vi "PXI_MultiTrig.vi"() -> ()   [LabVIEW 2018, in "Visualization.lvlib" / "VisualizeSync.lvclass"]
doc: "This VI listens for any measurement data associated with the provided PluginName and displays it to the user for analysis. The display is only suitable for data coming from the RoomAlert Plugin."
uses:
  VisualizeSync.lvclass
  VisualizeBase/VisualizeBase_class/SubVIs/VisualizationOptions.ctl
  <vilib>/Utility/miscctls.llb/LVRectTypeDef.ctl
  <vilib>/event_ctls.llb/usereventprio.ctl
  VisualizeBase/VisualizeBase_class/Requests/VisUserEventType.ctl
  <extravilib>/ChannelInstances/Tag-bool/Write With Abort.vi
  <extravilib>/ChannelInstances/Tag-bool/Read With Abort.vi
  <extravilib>/ChannelInstances/Tag-bool/Instantiate.vi
  <extravilib>/ChannelInstances/Tag-bool/EndpointRead.vi
  <vilib>/Utility/error.llb/Error Cluster From Error Code.vi
  <extravilib>/ChannelInstances/Tag-bool/Endpoint.vi
  <vilib>/ErrorRing/Error Ring.xnode
  <userlib>/NIST/NISTErrorLib/NISTErrorLib.lvlib
  VisualizeBase/VisualizeBase_class/VisualizeBase.lvclass
  <extravilib>/ChannelInstances/Tag-bool.lvlib
  TestClass/Test.lvclass
  Sync/SyncModule/SyncModule.lvlib
  StatusAndLog/VisualizeStatus.lvclass
panel:
  in  "btnPause":bool=TRUE
  in  "INIFilePath":path
  out "VisualizationProperties":T1={"PauseAtStartup"=TRUE, "LogData"=FALSE, "LaunchInSubPanel"=TRUE, "FPMonitor"=0, "FPWindowBounds"={"Left"=0, "Top"=0, "Right"=0, "Bottom"=0}, "MonitorBounds"={"Left"=0, "Top"=0, "Right"=0, "Bottom"=0}}
  in  "ModuleID":i32
  in  "Log Data":bool=TRUE
  in  "btnStop":bool
  in  "btnReset":bool
  in  "btnClearTest":bool
  out "LockStatus":bool
  out "Time Ref Offset (ns)":waveform(dbl)(graph)
  out "ErrorArray":errorcluster[](array[cluster])
  in  "PluginName":string="Sensor.RoomAlert1"
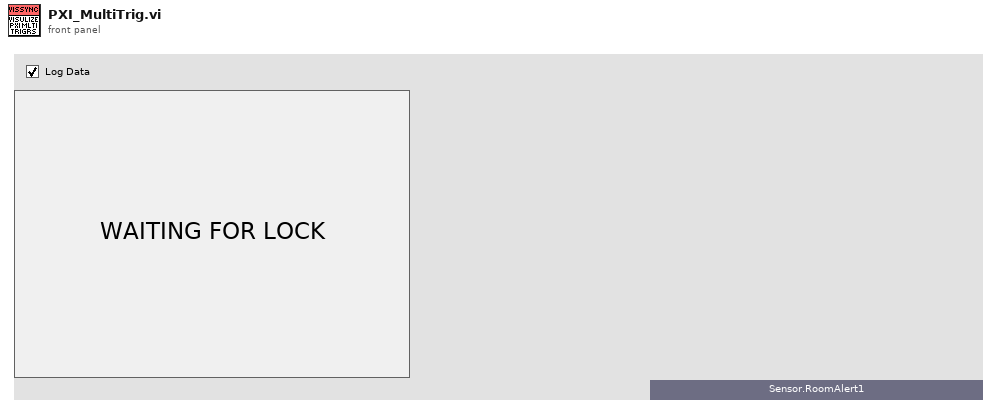
[diagram p1: front panel]
types:
  T1 = typedef "Visualization.lvlib/VisualizeBase.lvclass/VisualizationOptions.ctl" = cluster{"PauseAtStartup":bool, "LogData":bool, "LaunchInSubPanel":bool, "FPMonitor":u16, "FPWindowBounds":T2, "MonitorBounds":cluster{"Left":i16, "Top":i16, "Right":i16, "Bottom":i16}}
  T2 = typedef "LVRectTypeDef.ctl" = cluster{"Left":i16, "Top":i16, "Right":i16, "Bottom":i16}
  T3 = enum16{"open", "open or create", "create or replace", "create", "open (read-only)"}
  T4 = typedef "Visualization.lvlib/VisualizeBase.lvclass/VisRequestEvents.ctl" = cluster{"StopRequest":refnum<user-event>, "ResetRequest":refnum<user-event>, "FP Pop In or Out":refnum<user-event>}
  T5 = typedef "SyncModule.lvlib/SyncBroadcastEvents.ctl" = cluster{"DidInit":refnum<user-event>, "StatusUpdate":refnum<user-event>, "ErrorReport":refnum<user-event>, "DidStop":refnum<user-event>, "PathToINI":refnum<user-event>, "TriggerTime":refnum<user-event>, "LockStatus":refnum<user-event>, "Info":refnum<user-event>, "ClockProperties":refnum<user-event>, "SyncData":refnum<user-event>}
  T6 = cluster{"seconds since 1Jan1904":timestamp, "Time Ref Offset (ns)":dbl, "Lock":bool}
  T7 = typedef "Visualization.lvlib/VisualizeBase.lvclass/VisUserEventType.ctl" = cluster{"BusIndex":i8, "Data":variant}
  T8 = typedef "usereventprio.ctl" = enum32{"high priority", "normal priority"}
  T9 = typedef "Tag-bool.lvlib/))Channel.ctl" = refnum<queue>
  T10 = typedef "sizeaction.ctl" = enum32{"Minimized", "Maximized", "Resized"}
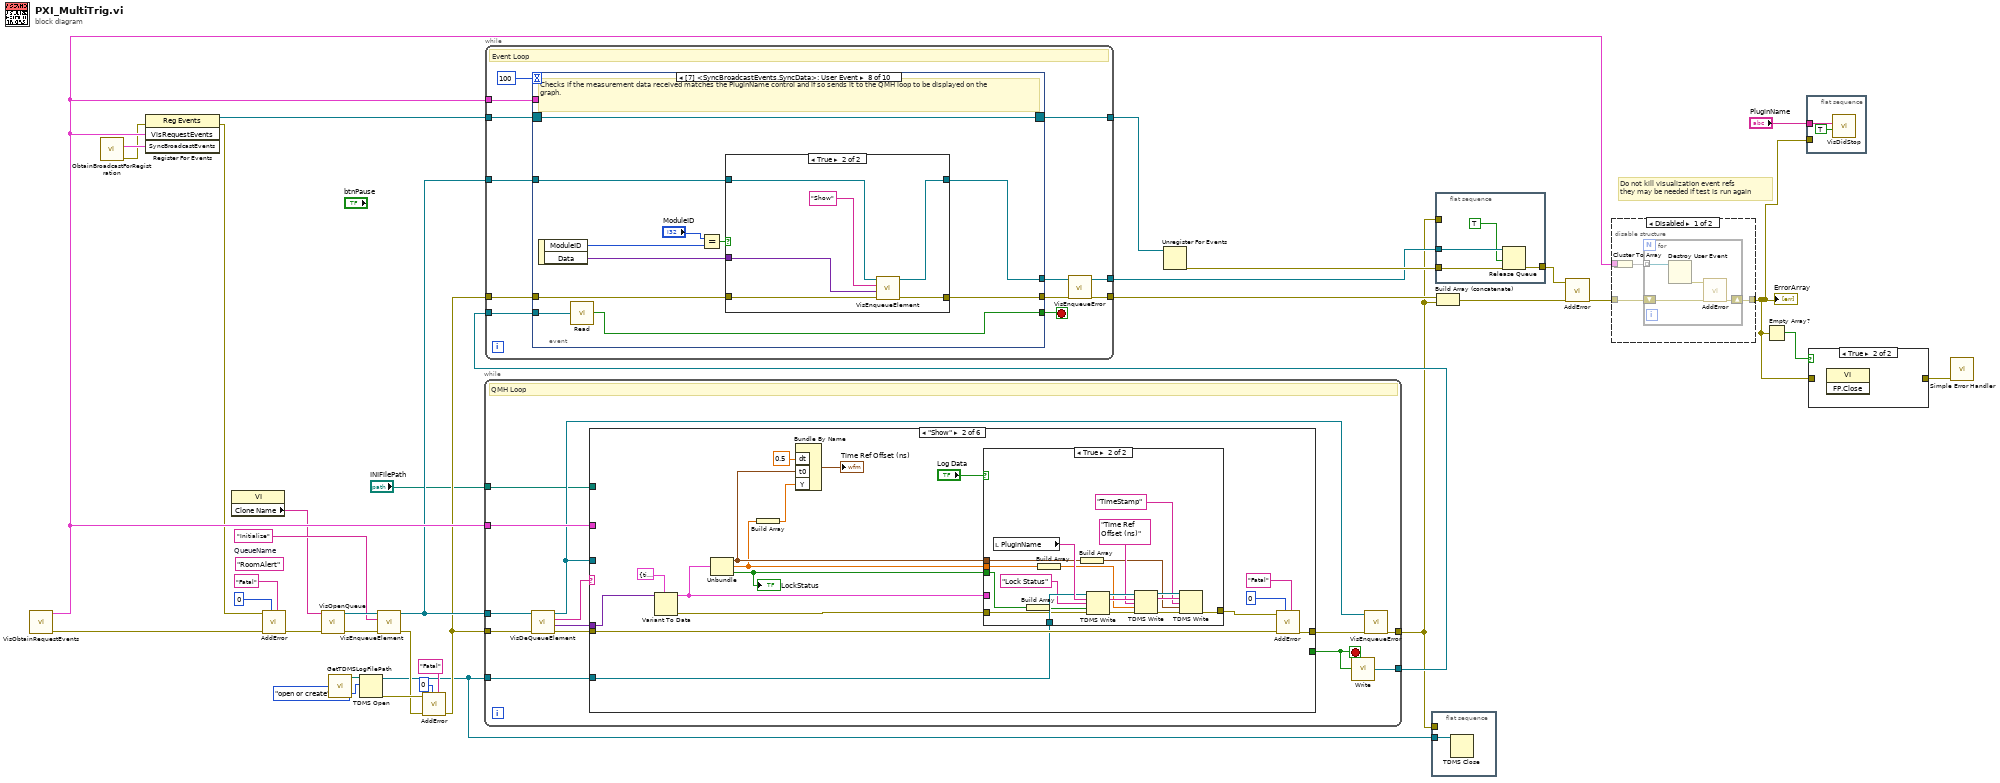
[diagram p0: block diagram]
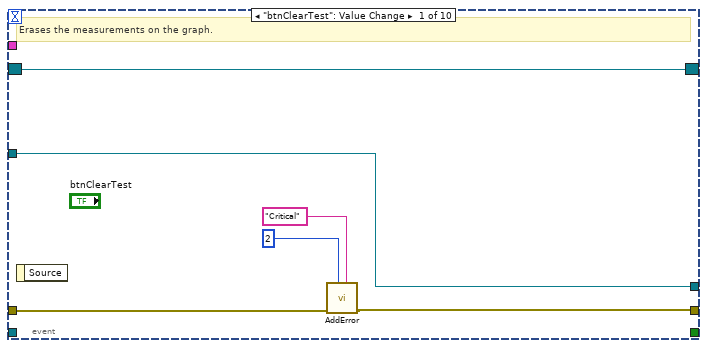
[diagram p3: hidden frame]
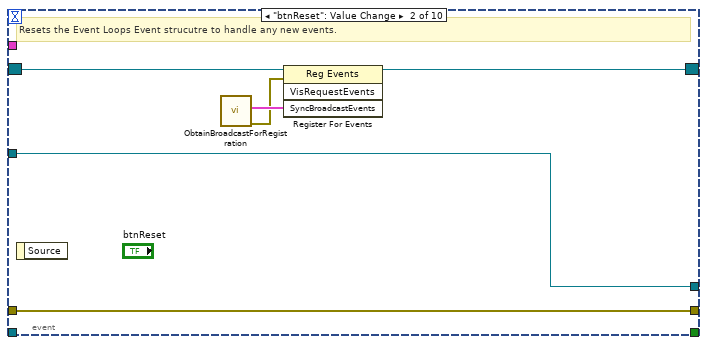
[diagram p4: hidden frame]
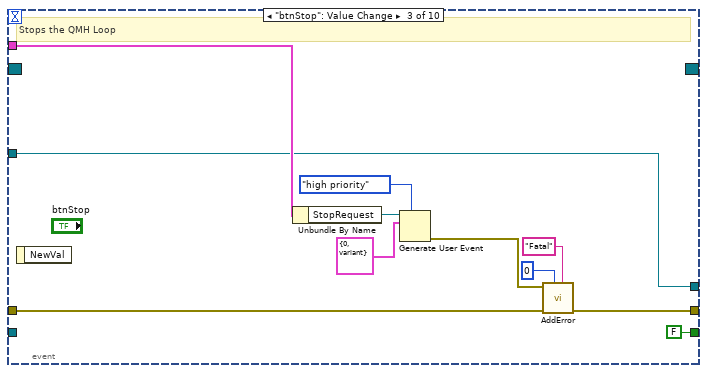
[diagram p5: hidden frame]
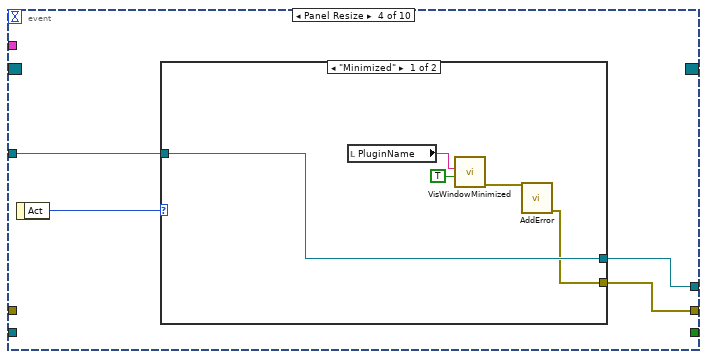
[diagram p6: hidden frame]
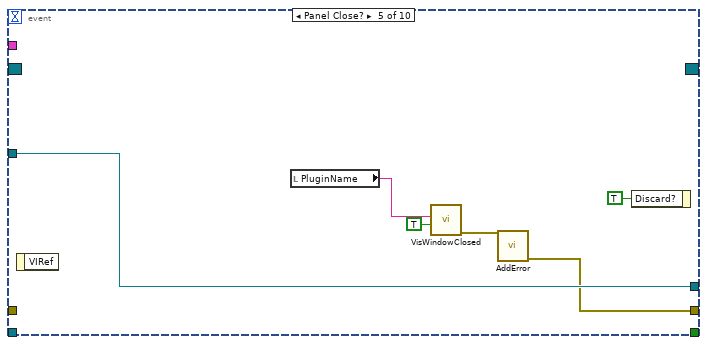
[diagram p8: hidden frame]
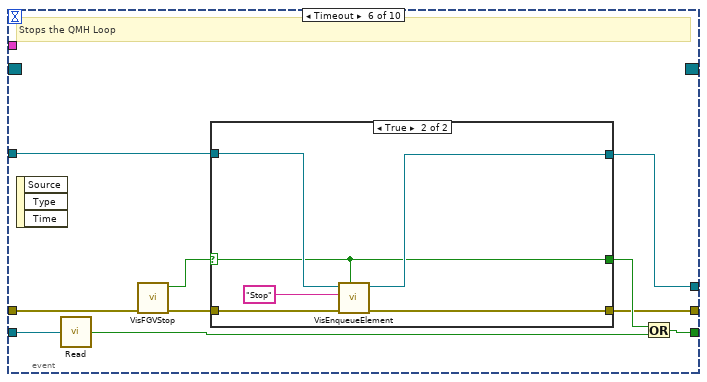
[diagram p9: hidden frame]
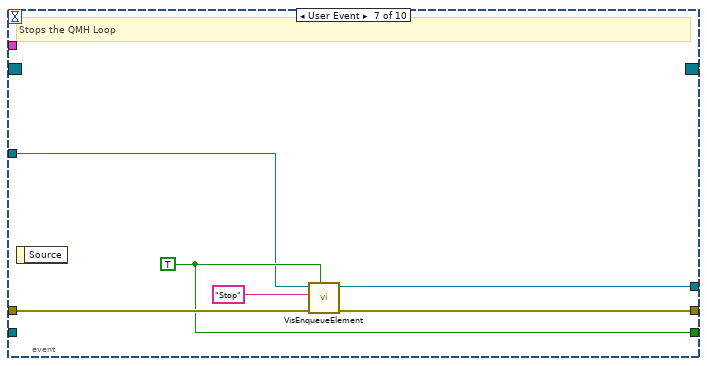
[diagram p11: hidden frame]
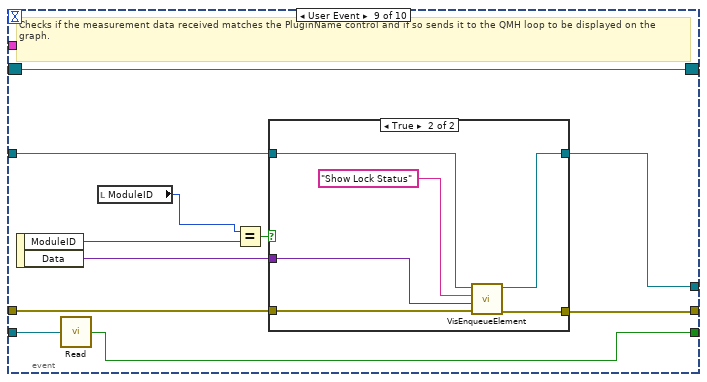
[diagram p13: hidden frame]
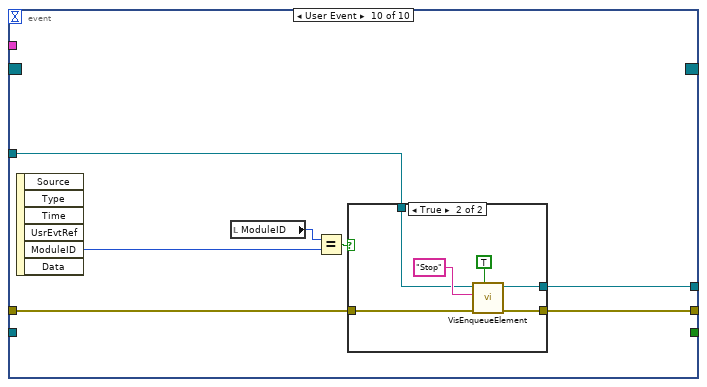
[diagram p15: hidden frame]
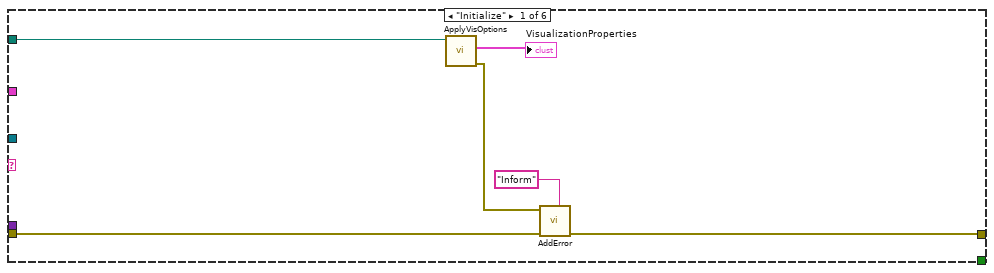
[diagram p17: hidden frame]
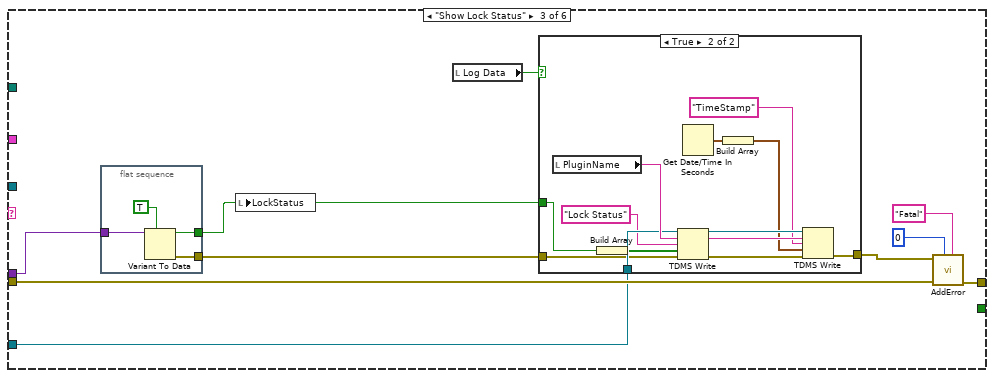
[diagram p19: hidden frame]
diagram:
  (unwired) "RoomAlert"  # QueueName
  # "Do not kill visualization event refs\nthey may be needed if test is run again"
  n1 = call "VisObtainRequestEvents.vi"() -> ("Error"=w27:errorcluster[], "VisRequestEvents"=w29:T4)  [unwired: 10 in]
  n2 = call "ObtainBroadcastForRegistration.vi"() -> ("error out"=w4:errorcluster, "SyncBroadcastEvents"=w5:T5)  [unwired: 10 in]
  n3 = register-events(error in=w4, w29, w5) -> (reference out=w36:refnum<event-registration>, error out=w26:errorcluster)  [unwired: 1 in]
  n4 = property class="VI"() -> ("Clone Name"=w15:string)  [unwired: 2 in, 2 out]
  n5 = call <userlib>:"AddError.vi"("Severity"="Fatal", "Priority"=u8 0, "ErrorArray In"=w27, "error in (no error)"=w26) -> ("ErrorArray Out"=w23:errorcluster[])  [unwired: 6 in, 1 out]
  n6 = call "VisOpenQueue.vi"("Error Array In"=w23, "QueueName"=w15) -> ("Error Array Out"=w21:errorcluster[], "queue out"=w22:refnum<queue>)  [unwired: 8 in]
  n7 = call "GetTDMSLogFilePath.vi"() -> ("TDMS Log File Path"=w14:path)  [unwired: 11 in]
  n8 = TDMS Open(10:T3."open or create" ("operation (0:open)"), 11:w14) -> (0:w11:errorcluster, 3:w7:refnum<k34>)  [unwired: 5 in]
  n9 = call "VisEnqueueElement.vi"("Error Array In"=w21, "Message"="Initialize", "queue in"=w22) -> ("Error Array Out"=w10:errorcluster[], "queue out"=w19:refnum<queue>)  [unwired: 7 in]
  n10 = call <userlib>:"AddError.vi"("Severity"="Fatal", "Priority"=u8 0, "ErrorArray In"=w10, "error in (no error)"=w11) -> ("ErrorArray Out"=w9:errorcluster[])  [unwired: 6 in, 1 out]
  n11 = while {
    tunnel: w9 -> [w43]
    tunnel: [w46] -> w6
    tunnel: w19 -> [w42]
    tunnel: w29 -> [w48]
    tunnel: [w39] -> w16
    tunnel: w7 -> [w38]
    tunnel: "INIFilePath" -> [w37]
    stop <- w49 stop-if-true
    # "QMH Loop"
    n12 = call "VisDeQueueElement.vi"("Error Array In"=w43, "Queue In"=w42) -> ("Error Array Out"=w41:errorcluster[], "Data"=w44:variant, "Message"=w45:string, "Queue Out"=w40:refnum<queue>)  [unwired: 6 in]
    n13 = case shown="\"Show\"" w45 {
      selector: w45 -> [_ _ _ w127 _ _]
      tunnel: w44 -> [_ w68 w98 _ w146 _]
      tunnel: w41 -> [w53 w71 w101 w125 _ w175]
      tunnel: [w52 w72 w102 w124 w136 w174] -> w47
      tunnel: [_ _ _ _ w142 TRUE] -> w49
      tunnel: w48 -> [_ _ _ _ w141 _]
      tunnel: w40 -> [_ _ _ _ w140 _]
      tunnel: w38 -> [_ w64 w95 _ _ _]
      tunnel: w37 -> [w51 _ _ _ _ w173]
      frame "Initialize" {
        n14 = call "ApplyVisOptions.vi"("INIFilePath"=w51) -> ("error out"=w54:errorcluster, "VisualizationProperties"=→"VisualizationProperties":T1)  [unwired: 9 in]
        n15 = call <userlib>:"AddError.vi"("Severity"="Inform", "ErrorArray In"=w53, "error in (no error)"=w54) -> ("ErrorArray Out"=w52:errorcluster[])  [unwired: 7 in, 1 out]
      }
      frame "Show" {
        n16 = Variant To Data(type=T6 {"seconds since 1Jan1904"=timestamp(0 s since 1904-01-01), "Time Ref Offset (ns)"=0.0, "Lock"=FALSE} ("output cluster"), Variant=w68) -> (data=w62:T6, error out=w67:errorcluster)  [unwired: 1 in]
        n17 = Unbundle(w62) -> ("seconds since 1Jan1904"=w59:timestamp, "Time Ref Offset (ns)"=w57:dbl, "Lock"=w60:bool)
        "LockStatus" <- w60
        n18 = Build Array(w57) -> (w61:dbl[])
        n19 = Bundle By Name("dt"=0.5, "t0"=w59, "Y"=w61) -> (→"Time Ref Offset (ns)":waveform(dbl))  [unwired: 1 in]
        n20 = case shown="True" "Log Data" {
          tunnel: w67 -> [w73 w90]
          tunnel: [w73 w79] -> w66
          tunnel: w64 -> [_ w91]
          tunnel: w62 -> [_ _]
          tunnel: w60 -> [_ w88]
          tunnel: w57 -> [_ w83]
          tunnel: w59 -> [_ w76]
          frame False {
          }
          frame True {
            n21 = local read "PluginName"() -> (w92:string)
            n22 = Build Array(w88) -> (w89:bool[])
            n23 = Build Array(w83) -> (w74:dbl[])
            n24 = Build Array(w76) -> (w75:timestamp[])
            n25 = TDMS Write(0:w91, 5:w92, 7:"Lock Status" ("PluginName"), 9:w89, 11:w90) -> (4:w86:refnum<k34>, 6:w85:string, 15:w84:errorcluster)  [unwired: 1 in, 1 out]
            n26 = TDMS Write(0:w86, 5:w85, 7:"Time Ref Offset (ns)" ("PluginName"), 9:w74, 11:w84) -> (4:w82:refnum<k34>, 6:w81:string, 15:w80:errorcluster)  [unwired: 1 in, 1 out]
            n27 = TDMS Write(0:w82, 5:w81, 7:"TimeStamp" ("PluginName"), 9:w75, 11:w80) -> (15:w79:errorcluster)  [unwired: 1 in, 3 out]
          }
        }
        n28 = call <userlib>:"AddError.vi"("Severity"="Fatal" ("String"), "Priority"=u8 0, "ErrorArray In"=w71, "error in (no error)"=w66) -> ("ErrorArray Out"=w72:errorcluster[])  [unwired: 6 in, 1 out]
      }
      frame "Show Lock Status" {
        n29 = flat-sequence {
          tunnel: w98 -> [w106]
          tunnel: [w105] -> w97
          tunnel: [w103] -> w93
          frame #0 {
            n30 = Variant To Data(type=TRUE, Variant=w106) -> (data=w103:bool, error out=w105:errorcluster)  [unwired: 1 in]
          }
        }
        n31 = local write "LockStatus"(w93) -> ()
        n32 = local read "Log Data"() -> (w94:bool)
        n33 = case shown="True" w94 {
          tunnel: w97 -> [w107 w118]
          tunnel: [w107 w111] -> w96
          tunnel: w95 -> [_ w119]
          tunnel: w93 -> [_ w116]
          frame False {
          }
          frame True {
            n34 = local read "PluginName"() -> (w120:string)
            n35 = Build Array(w116) -> (w117:bool[])
            n36 = TDMS Write(0:w119, 5:w120, 7:"Lock Status" ("PluginName"), 9:w117, 11:w118) -> (4:w114:refnum<k34>, 6:w113:string, 15:w112:errorcluster)  [unwired: 1 in, 1 out]
            n37 = Get Date/Time In Seconds() -> (seconds since 1Jan1904=w108:timestamp)
            n38 = Build Array(w108) -> (w109:timestamp[])
            n39 = TDMS Write(0:w114, 5:w113, 7:"TimeStamp" ("PluginName"), 9:w109, 11:w112) -> (15:w111:errorcluster)  [unwired: 1 in, 3 out]
          }
        }
        n40 = call <userlib>:"AddError.vi"("Severity"="Fatal" ("String"), "Priority"=u8 0, "ErrorArray In"=w101, "error in (no error)"=w96) -> ("ErrorArray Out"=w102:errorcluster[])  [unwired: 6 in, 1 out]
      }
      frame Default {
        n41 = xnode "Error Ring"("parameter 0"=w127) -> ("error out"=w126:errorcluster)
        n42 = call <userlib>:"AddError.vi"("Severity"="Inform" ("String"), "Priority"=u8 5, "ErrorArray In"=w125, "error in (no error)"=w126) -> ("ErrorArray Out"=w124:errorcluster[], "error out"=w123:errorcluster)  [unwired: 6 in]
        n43 = call <vilib>:"Clear Errors.vi"("error in (no error)"=w123) -> ()  [unwired: 5 in, 2 out]
      }
      frame "Error" {
        n44 = Variant To Data(type=errorcluster[] [], Variant=w146) -> (data=w144:errorcluster[], error out=w135:errorcluster)  [unwired: 1 in]
        n45 = call <userlib>:"ParseErrors.vi"("ErrorArray"=w144) -> ("ErrorArray"=w143:errorcluster[])  [unwired: 8 in, 2 out]
        n46 = for {
          tunnel: w143 -> [w157] mode=indexing
          tunnel: [w151] -> w137 mode=concatenating
          tunnel: [w149] -> w142
          tunnel: w141 -> [w148]
          tunnel: w140 -> [w147]
          stop <- w149 stop-if-true
          n47 = call <userlib>:"GeneralHandler.vi"("error in (no error)"=w157) -> ("Severity"=w150:string, "Stop"=w154:bool, "Abort"=w155:bool, "Continue"=w156:bool)  [unwired: 6 in, 1 out]
          n48 = Build Array(w156, w155, w154) -> (w153:bool[])
          n49 = Boolean Array To Number(Boolean array=w153) -> (number=w152:u32)
          n50 = case shown="1" w152 {
            tunnel: [_ _ w162 w171] -> w151
            tunnel: w150 -> [_ _ _ w164]
            tunnel: [_ _ _ w166] -> w149
            tunnel: w148 -> [_ _ _ w165]
            tunnel: w147 -> [_ _ w158 _]
            frame 0, Default {
              # "No Dialog"
            }
            frame 1 {
              # "Continue"
            }
            frame 2 {
              # "Abort, Flush Queue"
              n51 = Flush Queue(queue=w158) -> (error out=w161:errorcluster)  [unwired: 1 in, 2 out]
              n52 = call <userlib>:"AddError.vi"("Severity"="Critical" ("String"), "Priority"=u8 1, "error in (no error)"=w161) -> ("ErrorArray Out"=w162:errorcluster[])  [unwired: 7 in, 1 out]
            }
            frame 4 {
              # "Stop"
              n53 = Unbundle By Name(w165) -> ("StopRequest"=w172:refnum<user-event>)
              n54 = Equal?(x=w164, y="Fatal" ("x")) -> (x = y?=w166:bool)
              n55 = Generate User Event(priority (normal)=usereventprio."high priority", user event=w172, event data cluster=T7 {"BusIndex"=0, "Data"=variant} ("event data")) -> (error out=w170:errorcluster)  [unwired: 1 in, 1 out]
              n56 = call <userlib>:"AddError.vi"("error in (no error)"=w170) -> ("ErrorArray Out"=w171:errorcluster[], "error out"=w167:errorcluster)  [unwired: 9 in]
              n57 = call <vilib>:"Clear Errors.vi"("error in (no error)"=w167) -> ()  [unwired: 5 in, 2 out]
            }
          }
        }
        n58 = call <userlib>:"AddError.vi"("Severity"="Critical", "Priority"=u8 2, "ErrorArray In"=w137, "error in (no error)"=w135) -> ("ErrorArray Out"=w136:errorcluster[])  [unwired: 6 in, 1 out]
      }
      frame "Stop" {
        n59 = local read "VisualizationProperties"() -> (w176:T1)
        n60 = call "WriteVisOptionsToINIFile.vi"("Visualization Options"=w176, "INIFilePath"=w173) -> ("error out"=w178:errorcluster)  [unwired: 8 in, 1 out]
        n61 = call <userlib>:"AddError.vi"("Severity"="Inform", "ErrorArray In"=w175, "error in (no error)"=w178) -> ("ErrorArray Out"=w174:errorcluster[])  [unwired: 7 in, 1 out]
      }
    }
    n62 = call <extravilib>:"Write.vi"("element"=w49) -> ("channel"=w39:T9)  [unwired: 1 out]
    n63 = call "VisEnqueueError.vi"("Error Array In"=w47, "Queue in"=w40) -> ("Error Array Out"=w46:errorcluster[])  [unwired: 8 in, 1 out]
  }
  n64 = while {
    tunnel: w36 -> [w191]
    tunnel: [w185] -> w34
    tunnel: [w189] -> w35
    tunnel: w29 -> [w188]
    tunnel: w9 -> [w187]
    tunnel: w19 -> [w186]
    tunnel: [w182] -> w18
    tunnel: w16 -> [w180]
    stop <- w190 stop-if-true
    # "Event Loop"
    n65 = event shown="[7] <SyncBroadcastEvents.SyncData>: User Event" {
      selector: w191 -> [w193 w203 _ _ _ _ _ w262 w281 _]
      dyn-events: [w193 w202 _ _ _ _ _ w262 w281 _] -> w189
      timeout: 100 -> [_ _ _ _ _ _ _ _ _ _]
      tunnel: [_ _ FALSE ("Priority? (F)") _ _ w231 w252 w259 w278 _] -> w190
      tunnel: [w194 w201 w207 w217 w225 w233 w254 w264 w283 w298] -> w184
      tunnel: w188 -> [_ _ w206 _ _ _ _ _ _ _]
      tunnel: w187 -> [w195 w201 w214 _ _ w236 w255 w265 w284 w297]
      tunnel: w186 -> [w192 w200 w204 w216 w229 w235 w250 w266 w285 w296]
      tunnel: [w192 w200 w204 w215 w229 w234 w253 w263 w282 w299] -> w183
      tunnel: w180 -> [_ _ _ _ _ w240 _ w260 w279 _]
      event "btnClearTest": Value Change {
        # "Erases the measurements on the graph."
        n66 = event-data() -> ()  [unwired: 1 in, 1 out]
        n67 = call <userlib>:"AddError.vi"("Severity"="Critical", "Priority"=u8 2, "ErrorArray In"=w195) -> ("ErrorArray Out"=w194:errorcluster[])  [unwired: 7 in, 1 out]
      }
      event "btnReset": Value Change {
        # "Resets the Event Loops Event strucutre to handle any new events."
        n68 = event-data() -> ()  [unwired: 1 in, 1 out]
        n69 = call "ObtainBroadcastForRegistration.vi"() -> ("error out"=w198:errorcluster, "SyncBroadcastEvents"=w199:T5)  [unwired: 10 in]
        n70 = register-events(reference=w203, error in=w198, w199) -> (reference out=w202:refnum<event-registration>)  [unwired: 1 in, 1 out]
      }
      event "btnStop": Value Change {
        # "Stops the QMH Loop"
        n71 = event-data() -> ()  [unwired: 1 in, 1 out]
        n72 = Unbundle By Name(w206) -> ("StopRequest"=w212:refnum<user-event>)
        n73 = Generate User Event(priority (normal)=usereventprio."high priority", user event=w212, event data cluster=T7 {"BusIndex"=0, "Data"=variant} ("event data")) -> (error out=w213:errorcluster)  [unwired: 1 in, 1 out]
        n74 = call <userlib>:"AddError.vi"("Severity"="Fatal" ("String"), "Priority"=u8 0, "ErrorArray In"=w214, "error in (no error)"=w213) -> ("ErrorArray Out"=w207:errorcluster[])  [unwired: 6 in, 1 out]
      }
      event Panel Resize {
        n75 = event-data() -> ("Act"=w218:T10)  [unwired: 1 in]
        n76 = case shown="\"Minimized\"" w218 {
          tunnel: [w220 _] -> w217
          tunnel: w216 -> [w221 w224]
          tunnel: [w221 w224] -> w215
          frame "Minimized" {
            n77 = local read "PluginName"() -> (w223:string)
            n78 = call "VisWindowMinimized.vi"("Window Minimized?"=TRUE ("Window Minimized or Clozed?"), "Module Name"=w223) -> ("error out"=w222:errorcluster)  [unwired: 9 in]
            n79 = call <userlib>:"AddError.vi"("error in (no error)"=w222) -> ("ErrorArray Out"=w220:errorcluster[])  [unwired: 9 in, 1 out]
          }
          frame "Maximized", Default {
          }
        }
      }
      event Panel Close? {
        n80 = event-data() -> ()  [unwired: 1 in, 1 out]
        n81 = local read "PluginName"() -> (w228:string)
        n82 = call "VisWindowClosed.vi"("Window Closed?"=TRUE ("Window Minimized or Clozed?"), "Module Name"=w228) -> ("error out"=w227:errorcluster)  [unwired: 9 in]
        n83 = call <userlib>:"AddError.vi"("error in (no error)"=w227) -> ("ErrorArray Out"=w225:errorcluster[])  [unwired: 9 in, 1 out]
        n84 = event-data("Discard?"=TRUE) -> ()  [unwired: 1 in, 1 out]
      }
      event Timeout {
        # "Stops the QMH Loop"
        n85 = event-data() -> ()  [unwired: 1 in, 3 out]
        n86 = call <extravilib>:"Read.vi"("channel"=w240) -> ("element"=w232:bool)  [unwired: 1 in, 1 out]
        n87 = call "VisFGVStop.vi"("Error In"=w236) -> ("Error Out"=w238:errorcluster[], "Value"=w239:bool)  [unwired: 9 in]
        n88 = case shown="True" w239 {
          selector: w239 -> [w241 w244]
          tunnel: [w243 w247] -> w233
          tunnel: w238 -> [w243 w248]
          tunnel: w235 -> [w242 w246]
          tunnel: [w242 w245] -> w234
          tunnel: [w241 w244] -> w237
          frame False {
          }
          frame True {
            n89 = call "VisEnqueueElement.vi"("Priority? (F)"=w244, "Error Array In"=w248, "Message"="Stop", "queue in"=w246) -> ("Error Array Out"=w247:errorcluster[], "queue out"=w245:refnum<queue>)  [unwired: 6 in]
          }
        }
        n90 = Or(x=w237, y=w232) -> (x .or. y?=w231:bool)
      }
      event User Event {
        w252 = TRUE ("Priority? (F)")
        # "Stops the QMH Loop"
        n91 = event-data() -> ()  [unwired: 1 in, 1 out]
        n92 = call "VisEnqueueElement.vi"("Priority? (F)"=w252, "Error Array In"=w255, "Message"="Stop", "queue in"=w250) -> ("Error Array Out"=w254:errorcluster[], "queue out"=w253:refnum<queue>)  [unwired: 6 in]
      }
      event User Event {
        # "Checks if the measurement data received matches the PluginName control and if so sends it to the QMH loop to be displayed on the graph."
        n93 = event-data() -> ("ModuleID"=w257:i32, "Data"=w258:variant)  [unwired: 1 in]
        n94 = call <extravilib>:"Read.vi"("channel"=w260) -> ("element"=w259:bool)  [unwired: 1 in, 1 out]
        n95 = Equal?(x="ModuleID", y=w257) -> (x = y?=w261:bool)
        n96 = case shown="True" w261 {
          tunnel: [w267 w273] -> w264
          tunnel: w266 -> [w268 w272]
          tunnel: w265 -> [w267 w274]
          tunnel: [w268 w271] -> w263
          tunnel: w258 -> [_ w269]
          frame False {
          }
          frame True {
            n97 = call "VisEnqueueElement.vi"("Error Array In"=w274, "Data"=w269, "Message"="Show", "queue in"=w272) -> ("Error Array Out"=w273:errorcluster[], "queue out"=w271:refnum<queue>)  [unwired: 6 in]
          }
        }
      }
      event User Event {
        # "Checks if the measurement data received matches the PluginName control and if so sends it to the QMH loop to be displayed on the graph."
        n98 = event-data() -> ("ModuleID"=w276:i32, "Data"=w277:variant)  [unwired: 1 in]
        n99 = call <extravilib>:"Read.vi"("channel"=w279) -> ("element"=w278:bool)  [unwired: 1 in, 1 out]
        n100 = local read "ModuleID"() -> (w275:i32)
        n101 = Equal?(x=w275, y=w276) -> (x = y?=w280:bool)
        n102 = case shown="True" w280 {
          tunnel: [w286 w292] -> w283
          tunnel: w285 -> [w287 w291]
          tunnel: w284 -> [w286 w293]
          tunnel: [w287 w290] -> w282
          tunnel: w277 -> [_ w288]
          frame False {
          }
          frame True {
            n103 = call "VisEnqueueElement.vi"("Error Array In"=w293, "Data"=w288, "Message"="Show Lock Status", "queue in"=w291) -> ("Error Array Out"=w292:errorcluster[], "queue out"=w290:refnum<queue>)  [unwired: 6 in]
          }
        }
      }
      event User Event {
        n104 = event-data() -> ("ModuleID"=w294:i32)  [unwired: 1 in, 5 out]
        n105 = local read "ModuleID"() -> (w295:i32)
        n106 = Equal?(x=w295, y=w294) -> (x = y?=w300:bool)
        n107 = case shown="True" w300 {
          tunnel: [w301 w306] -> w298
          tunnel: [w302 w305] -> w299
          tunnel: w296 -> [w302 w304]
          tunnel: w297 -> [w301 w303]
          frame False {
          }
          frame True {
            n108 = call "VisEnqueueElement.vi"("Priority? (F)"=TRUE, "Error Array In"=w303, "Message"="Stop", "queue in"=w304) -> ("Error Array Out"=w306:errorcluster[], "queue out"=w305:refnum<queue>)  [unwired: 6 in]
          }
        }
      }
    }
    n109 = call "VisEnqueueError.vi"("Error Array In"=w184, "Queue in"=w183) -> ("Error Array Out"=w185:errorcluster[], "Queue out"=w182:refnum<queue>)  [unwired: 8 in]
  }
  n110 = Unregister For Events(event registration refnum=w35) -> (error out=w33:errorcluster)  [unwired: 1 in]
  n111 = flat-sequence {
    tunnel: w7 -> [w309]
    tunnel: w6 -> [_]
    frame #0 {
      n112 = TDMS Close(11:w309) -> ()  [unwired: 1 in, 2 out]
    }
  }
  n113 = flat-sequence {
    tunnel: w33 -> [w313]
    tunnel: [w312] -> w31
    tunnel: w18 -> [w311]
    tunnel: w6 -> [_]
    frame #0 {
      n114 = Release Queue(queue=w311, force destroy? (F)=TRUE, error in (no error)=w313) -> (error out=w312:errorcluster)  [unwired: 2 out]
    }
  }
  n115 = Build Array (concatenate)(w34, w6) -> (w32:errorcluster[])
  n116 = call <userlib>:"AddError.vi"("ErrorArray In"=w32, "error in (no error)"=w31) -> ("ErrorArray Out"=w30:errorcluster[])  [unwired: 8 in, 1 out]
  n117 = disable-structure shown="Disabled" {
    disable-tunnel: w30 -> [w316 w322]
    disable-tunnel: w29 -> [w315 _]
    disable-tunnel: [w314 w322] -> w2
    frame Disabled {
      n118 = Cluster To Array(cluster=w315) -> (array=w317:refnum<user-event>[])
      n119 = for {
        tunnel: w317 -> [w321] mode=indexing
        shift-right: [w320] -> w314
        shift-left: w316 -> [w319]
        n120 = Destroy User Event(user event=w321) -> (error out=w318:errorcluster)  [unwired: 1 in]
        n121 = call <userlib>:"AddError.vi"("ErrorArray In"=w319, "error in (no error)"=w318) -> ("ErrorArray Out"=w320:errorcluster[])  [unwired: 8 in, 1 out]
      }
    }
    frame Enabled {
    }
  }
  "ErrorArray" <- w2
  n122 = Empty Array?(array=w2) -> (empty?=w28:bool)
  n123 = flat-sequence {
    tunnel: "PluginName" -> [w324]
    tunnel: w2 -> [_]
    frame #0 {
      n124 = call "VisDidStop.vi"("DidStop?"=TRUE, "Module Name"=w324) -> ()  [unwired: 9 in, 1 out]
    }
  }
  n125 = case shown="True" w28 {
    tunnel: [w325 _] -> w17
    tunnel: w2 -> [w326 _]
    frame False {
      n126 = Merge Errors(w326) -> (w325:errorcluster)
    }
    frame True {
      n127 = invoke class="VI" method="FP.Close"() -> ()  [unwired: 3 in, 3 out]
    }
  }
  n128 = call <vilib>:"Simple Error Handler.vi"("error in (no error)"=w17) -> ()  [unwired: 4 in, 5 out]
